vi "Actor Core.vi"(8 "error in (no error)":errorcluster, 11 "Operator UI.lvclass":refnum<class "Server UI.lvclass">) -> (0 "error out":errorcluster, 3 "Actor Framework.lvlib:Actor":refnum<class "Actor.lvclass">)   [LabVIEW 2017, in "Server UI.lvlib" / "Server UI.lvclass"]
doc: "This is Actor Core.vi, the main message handling loop for Actors. An actor usually just sits in this loop and processes messages as they arrive. Any error returned by the message Do.vi call will stop the loop, with error code 43 as the cannonical signal to stop with no error sent to caller. Descendants may override that in Handle Error.vi."
uses:
  Server UI.lvclass
  <vilib>/ActorFramework/Actor/Actor.lvclass
  \\Mac\Home/Documents/MAL-Framework/user.lib/Common Components/Msmt UI/Measurement UI.lvclass
  \\Mac\Home/Documents/MAL-Framework/user.lib/Common Components/User Interface/UI.lvclass
  C:/Program Files (x86)/National Instruments/LabVIEW 2017/vi.lib/ActorFramework/Actor/Actor.lvclass
  Server UI.lvclass/Server UI.ctl
  <vilib>/ActorFramework/Actor/Actor.lvclass/Actor.ctl
  <vilib>/ActorFramework/Message Enqueuer/Message Enqueuer.lvclass/Message Enqueuer.ctl
  Write Start Server.vi
  Write Connected Clients.vi
  <vilib>/ActorFramework/Message Enqueuer/Init from Existing Queue.vi
  <vilib>/ActorFramework/Message Enqueuer/Enqueue.vi
  <vilib>/ActorFramework/Stop Msg/Stop Msg.lvclass
  C:/Program Files (x86)/National Instruments/LabVIEW 2017/vi.lib/ActorFramework/Message/Message.lvclass
  MAL-Framework/user.lib/Common Components/User Interface/Messages/Disable UI Msg/Disable UI Msg.lvclass
  Server UI Messages/Show Connections Msg/Show Connections Msg.lvclass
  MAL-Framework/user.lib/Common Components/Msmt UI/Messages/Ask Controller to Launch Results UI Msg/Ask Controller to Launch Results UI Msg.lvclass
  MAL-Framework/user.lib/Common Components/User Interface/Messages/Reset Controls Msg/Reset Controls Msg.lvclass
  Server UI Messages/Reset Measurement List Display Msg/Reset Measurement List Display Msg.lvclass
  MAL-Framework/user.lib/Common Components/Measurement UI Messages/Launch Step Configuration Msg/Launch Step Configuration Msg.lvclass
  MAL-Framework/user.lib/Common Components/User Interface/Messages/Enable UI Msg/Enable UI Msg.lvclass
  MAL-Framework/user.lib/Common Components/Msmt UI/Messages/Tell Controller to Launch Settings Dialog Msg/Tell Controller to Launch Settings Dialog Msg.lvclass
  MAL-Framework/user.lib/Common Components/Msmt UI/Accessors/Write Digitizer.vi
  MAL-Framework/user.lib/Common Components/Msmt UI/Accessors/Write Function Generator.vi
  MAL-Framework/user.lib/Common Components/Msmt UI/Accessors/Write Load New Measurement.vi
  MAL-Framework/user.lib/Common Components/Msmt UI/Accessors/Write Measurement.vi
  MAL-Framework/user.lib/Common Components/Msmt UI/Accessors/Write Multimeter.vi
  MAL-Framework/user.lib/Common Components/Msmt UI/Accessors/Write Power Supply.vi
  MAL-Framework/user.lib/Common Components/Msmt UI/Accessors/Write Results Listbox.vi
  MAL-Framework/user.lib/Common Components/Msmt UI/Accessors/Write Run.vi
  MAL-Framework/user.lib/Common Components/Msmt UI/Accessors/Write Show FP_.vi
  MAL-Framework/user.lib/Common Components/Msmt UI/Accessors/Write Status Display.vi
  MAL-Framework/user.lib/Common Components/Msmt UI/Accessors/Write Tab Control.vi
  MAL-Framework/user.lib/Common Components/Msmt UI/Accessors/Write View Results.vi
  MAL-Framework/user.lib/Common Components/User Interface/Accessors/Write Settings Button.vi
  MAL-Framework/user.lib/Common Components/Msmt UI/Accessors/Write Run Indefinitely.vi
  MAL-Framework/user.lib/Common Components/Msmt UI/Write Step Iterations.vi
  MAL-Framework/user.lib/Common Components/Msmt UI/Write settings button array for hardware.vi
  MAL-Framework/user.lib/Common Components/Msmt UI/Accessors/Write Step Config.vi
  <vilib>/ActorFramework/Message Priority Queue/Priority Enqueue.vi
  <vilib>/ActorFramework/Message Enqueuer/Message Enqueuer.lvclass
  MAL-Framework/user.lib/Common Components/Msmt UI/Measurement UI.lvclass
  MAL-Framework/user.lib/Common Components/Msmt UI/Messages/Send Run Measurement Message/Send Run Measurement Message.lvclass
  MAL-Framework/user.lib/Common Components/Msmt UI/Messages/Send Get Hardware Info Message/Send Get Hardware Info Message.lvclass
  MAL-Framework/user.lib/Common Components/Msmt UI/Messages/Check Run Button/Check Validity of Selection.lvclass
  MAL-Framework/user.lib/Common Components/Msmt UI/Messages/Prompt User for Path to load/Prompt User for File Path to Load From.lvclass
  MAL-Framework/user.lib/Common Components/User Interface/UI.lvclass
  MAL-Framework/user.lib/Common Components/Measurement UI Messages/Launch Hardware Settings Msg/Launch Hardware Settings Msg.lvclass
panel:
  in  "Connected Clients":i32(listbox)
  in  "Step Config":bool
  in  "3":bool
  in  "2":bool
  in  "1":bool
  in  "0":bool
  in  "Step Iterations":i32
  in  "Run Indefinitely":bool
  in  "Show FP?":bool
  in  "Power Supply":u16(ring) caption="4"
  in  "Function Generator":u16(ring) caption="3"
  in  "Digitizer":u16(ring) caption="2"
  in  "Multimeter":u16(ring) caption="1"
  in  "Step":u16(ring)
  in  "about":bool
  in  "Tab Control":enum32{"Test Status", "Results"}(tab)
  in  "Status Display":string
  in  "View Results":bool
  in  "Results Listbox":i32(listbox)
  in  "Settings Button":bool
  in  "Start Server":bool
  in  "Load New Measurement":bool
  in  "Run":bool
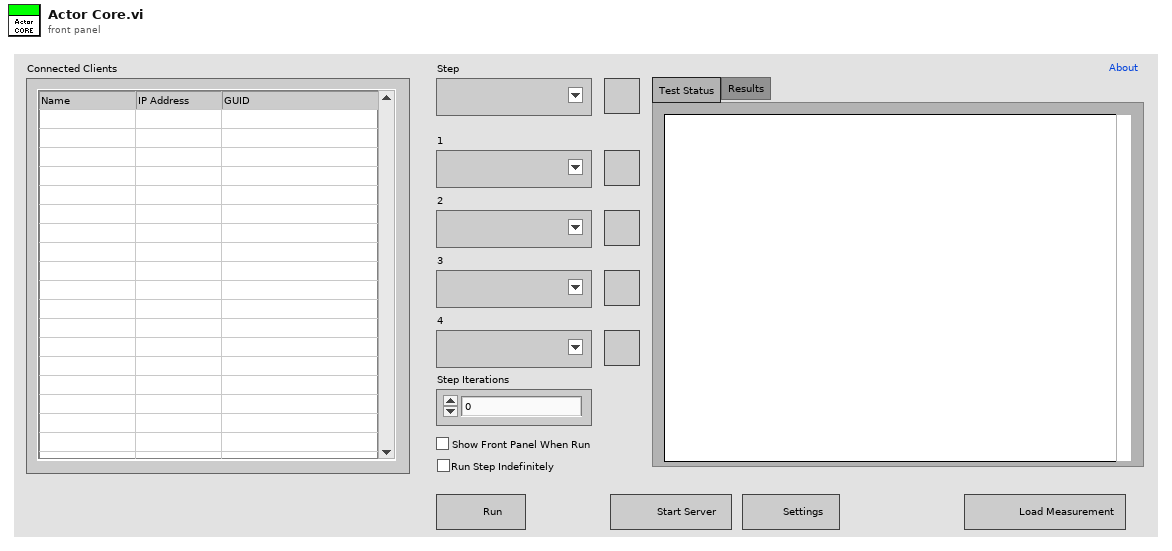
[diagram p1: front panel]
types:
  T1 = enum8{"Enabled", "Disabled", "Disabled and Grayed Out"}
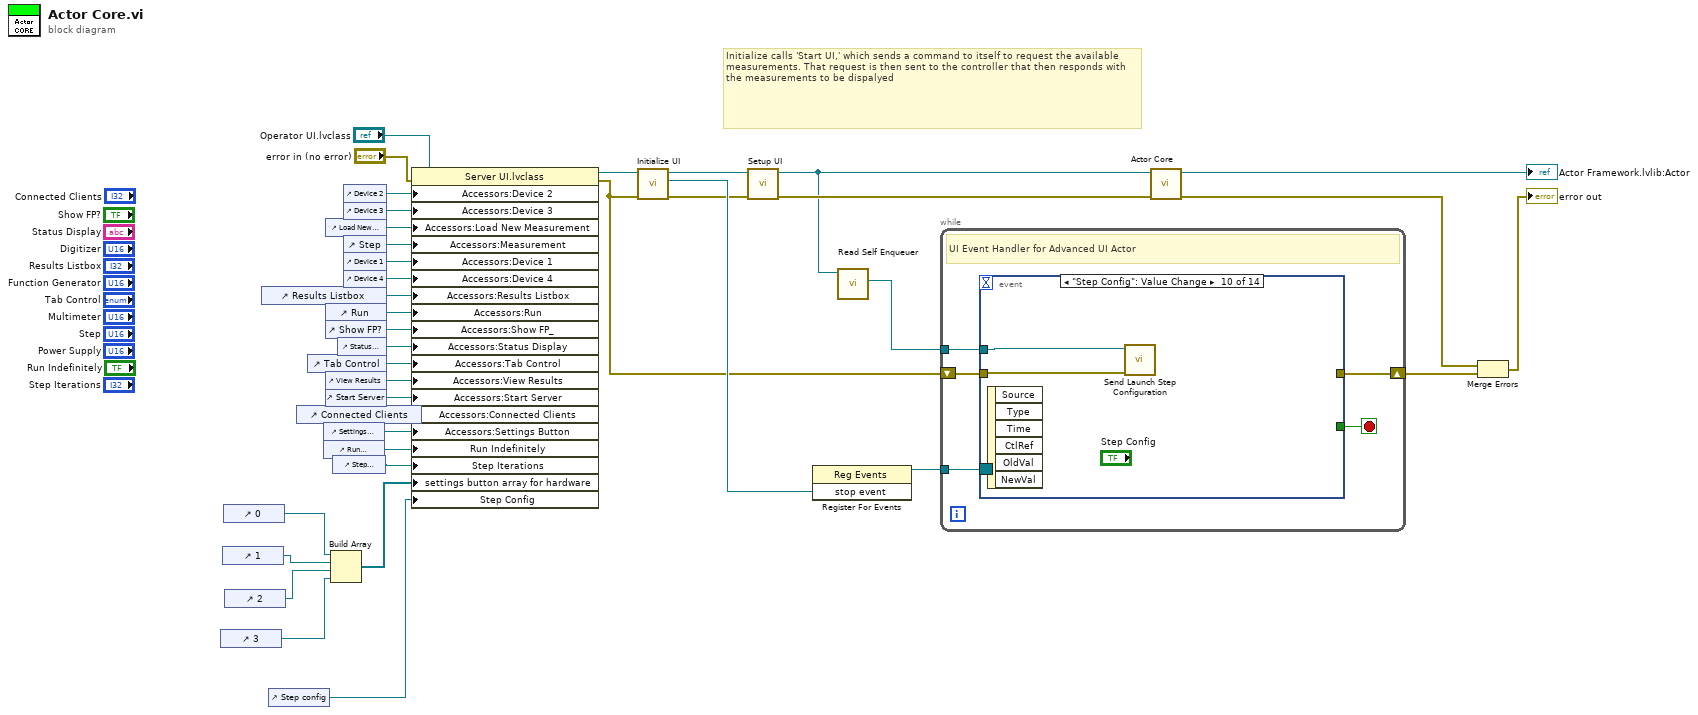
[diagram p0: block diagram]
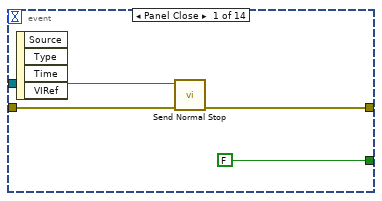
[diagram p2: hidden frame]
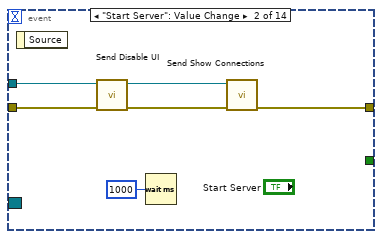
[diagram p3: hidden frame]
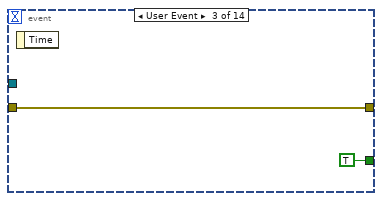
[diagram p4: hidden frame]
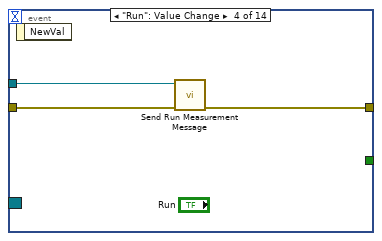
[diagram p5: hidden frame]
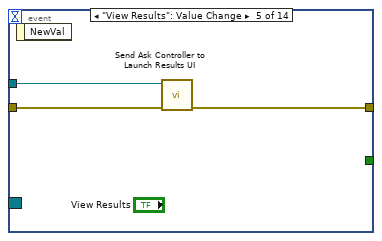
[diagram p6: hidden frame]
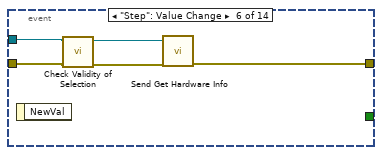
[diagram p7: hidden frame]
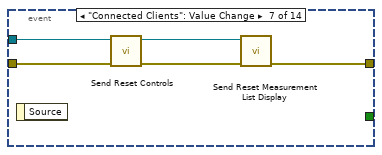
[diagram p8: hidden frame]
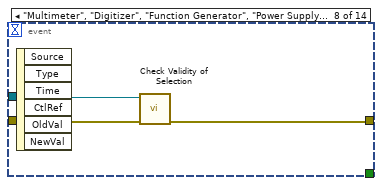
[diagram p9: hidden frame]
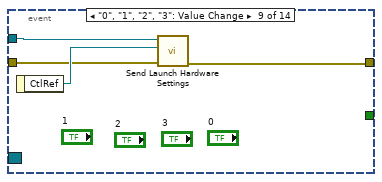
[diagram p10: hidden frame]
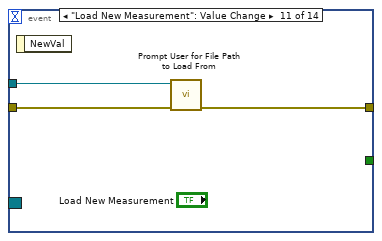
[diagram p11: hidden frame]
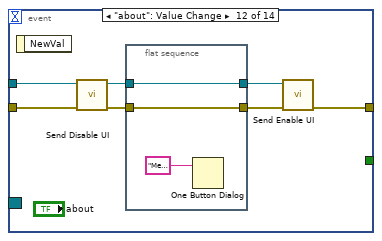
[diagram p12: hidden frame]
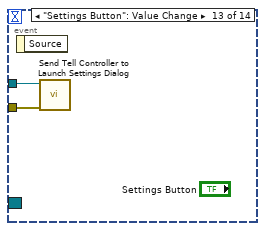
[diagram p13: hidden frame]
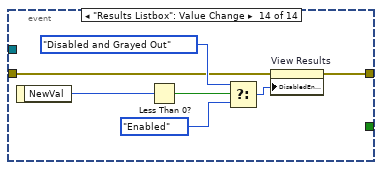
[diagram p14: hidden frame]
diagram:
  # "Initialize calls 'Start UI,' which sends a command to itself to request the available measurements. That request is then sent to the controller that then responds with the measurements to be dispalyed"
  n1 = control-ref of="3"() -> (w6:refnum<vi>)
  n2 = control-ref of="1"() -> (w4:refnum<vi>)
  n3 = control-ref of="0"() -> (w3:refnum<vi>)
  n4 = control-ref of="2"() -> (w5:refnum<vi>)
  n5 = control-ref of="Results Listbox"() -> (w29:refnum<vi>)
  n6 = control-ref of="Step config"() -> (w1:refnum<vi>)
  n7 = control-ref of="Connected Clients"() -> (w11:refnum<vi>)
  n8 = control-ref of="Tab Control"() -> (w31:refnum<vi>)
  n9 = control-ref of="Settings Button"() -> (w9:refnum<vi>)
  n10 = control-ref of="Run Indefinitely"() -> (w8:refnum<vi>)
  n11 = control-ref of="Load New Measurement"() -> (w25:refnum<vi>)
  n12 = control-ref of="Run"() -> (w22:refnum<vi>)
  n13 = control-ref of="Show FP?"() -> (w33:refnum<vi>)
  n14 = control-ref of="View Results"() -> (w30:refnum<vi>)
  n15 = control-ref of="Start Server"() -> (w12:refnum<vi>)
  n16 = Build Array(w3, w4, w5, w6) -> (w2:refnum<vi>[])
  n17 = control-ref of="Step Iterations"() -> (w7:refnum<vi>)
  n18 = control-ref of="Status Display"() -> (w32:refnum<vi>)
  n19 = control-ref of="Device 2"() -> (w27:refnum<vi>)
  n20 = control-ref of="Device 3"() -> (w26:refnum<vi>)
  n21 = control-ref of="Step"() -> (w24:refnum<vi>)
  n22 = control-ref of="Device 1"() -> (w23:refnum<vi>)
  n23 = control-ref of="Device 4"() -> (w28:refnum<vi>)
  n24 = property class="Server UI.lvclass"(reference="Operator UI.lvclass", error in="error in (no error)", "Accessors:Device 2"=w27, "Accessors:Device 3"=w26, "Accessors:Load New Measurement"=w25, "Accessors:Measurement"=w24, "Accessors:Device 1"=w23, "Accessors:Device 4"=w28, "Accessors:Results Listbox"=w29, "Accessors:Run"=w22, "Accessors:Show FP_"=w33, "Accessors:Status Display"=w32, "Accessors:Tab Control"=w31, "Accessors:View Results"=w30, "Accessors:Start Server"=w12, "Accessors:Connected Clients"=w11, "Accessors:Settings Button"=w9, "Run Indefinitely"=w8, "Step Iterations"=w7, "settings button array for hardware"=w2, "Step Config"=w1) -> (reference out=w17:refnum<class "Server UI.lvclass">, error out=w14:errorcluster)
  n25 = call "Initialize UI.vi"("error in (no error)"=w14, "UI in"=w17) -> ("error out"=w13:errorcluster, "stop event"=w34:refnum<user-event>, "UI out"=w16:refnum<class "Server UI.lvclass">)  [unwired: 7 in]
  n26 = call-dynamic "Setup UI.vi"("error in (no error)"=w13, "Operator UI in"=w16) -> ("error out"=w15:errorcluster, "Operator UI out"=w10:refnum<class "Server UI.lvclass">)  [unwired: 8 in]
  n27 = register-events(w34) -> (reference out=w35:refnum<event-registration>)  [unwired: 2 in, 1 out]
  n28 = call <vilib>:"Read Self Enqueuer.vi"("Actor"=w10) -> ("Self Enqueuer"=w37:refnum<class "Message Enqueuer.lvclass">)  [unwired: 10 in]
  n29 = while {
    tunnel: w37 -> [w42]
    tunnel: w35 -> [w41]
    shift-right: [w39] -> w36
    shift-left: w14 -> [w40]
    stop <- w43 stop-if-true
    # "UI Event Handler for Advanced UI Actor"
    n30 = event shown="[9] \"Step Config\": Value Change" {
      selector: w41 -> [_ _ _ _ _ _ _ _ _ _ _ _ _ _]
      dyn-events: _ -> [_ _ _ _ _ _ _ _ _ _ _ _ _ _]
      timeout: _ -> [_ _ _ _ _ _ _ _ _ _ _ _ _ _]
      tunnel: [FALSE _ TRUE _ _ _ _ _ _ _ _ _ _ _] -> w43
      tunnel: w42 -> [w46 w51 _ w58 w61 w65 w71 w74 w78 w80 w83 w90 w94 _]
      tunnel: w40 -> [w45 w50 w54 w57 w60 w64 w70 w73 w76 w79 w82 w89 w95 w97]
      tunnel: [w44 w48 w54 w56 w59 w66 w67 w72 w75 _ w81 w84 _ w96] -> w39
      event Panel Close {
        n31 = event-data() -> ()  [unwired: 1 in, 4 out]
        n32 = call <vilib>:"Send Normal Stop.vi"("error in (no error)"=w45, "Message Enqueuer"=w46) -> ("error out"=w44:errorcluster)  [unwired: 9 in]
      }
      event "Start Server": Value Change {
        n33 = event-data() -> ()  [unwired: 1 in, 1 out]
        n34 = call "Send Disable UI.vi"("error in (no error)"=w50, "Message Enqueuer"=w51) -> ("error out"=w49:errorcluster, "Message Enqueuer out"=w52:refnum<class "Message Enqueuer.lvclass">)  [unwired: 8 in]
        n35 = Wait (ms)(milliseconds to wait=u32 1000) -> ()  [unwired: 1 out]
        n36 = call "Send Show Connections.vi"("error in (no error)"=w49, "Message Enqueuer"=w52) -> ("error out"=w48:errorcluster)  [unwired: 8 in, 1 out]
      }
      event User Event {
        n37 = event-data() -> ()  [unwired: 1 in, 1 out]
      }
      event "Run": Value Change {
        n38 = event-data() -> ()  [unwired: 1 in, 1 out]
        n39 = call "Send Run Measurement Message.vi"("error in (no error)"=w57, "Message Enqueuer in"=w58) -> ("error out"=w56:errorcluster)  [unwired: 8 in, 1 out]
      }
      event "View Results": Value Change {
        n40 = event-data() -> ()  [unwired: 1 in, 1 out]
        n41 = call "Send Ask Controller to Launch Results UI.vi"("error in (no error)"=w60, "Message Enqueuer in"=w61) -> ("error out"=w59:errorcluster)  [unwired: 8 in, 1 out]
      }
      event "Step": Value Change {
        n42 = event-data() -> ()  [unwired: 1 in, 1 out]
        n43 = call "Check Validity of Selection.vi"("error in (no error)"=w64, "Message Enqueuer in"=w65) -> ("error out"=w63:errorcluster, "Message Enqueuer out"=w62:refnum<class "Message Enqueuer.lvclass">)  [unwired: 8 in]
        n44 = call "Send Get Hardware Info.vi"("error in (no error)"=w63, "Message Enqueuer in"=w62) -> ("error out"=w66:errorcluster)  [unwired: 8 in, 1 out]
      }
      event "Connected Clients": Value Change {
        n45 = event-data() -> ()  [unwired: 1 in, 1 out]
        n46 = call "Send Reset Controls.vi"("error in (no error)"=w70, "Message Enqueuer"=w71) -> ("error out"=w68:errorcluster, "Message Enqueuer out"=w69:refnum<class "Message Enqueuer.lvclass">)  [unwired: 8 in]
        n47 = call "Send Reset Measurement List Display.vi"("error in (no error)"=w68, "Message Enqueuer"=w69) -> ("error out"=w67:errorcluster)  [unwired: 8 in, 1 out]
      }
      event "Multimeter", "Digitizer", "Function Generator", "Power Supply", "Step Iterations", "Run Indefinitely": Value Change {
        n48 = event-data() -> ()  [unwired: 1 in, 6 out]
        n49 = call "Check Validity of Selection.vi"("error in (no error)"=w73, "Message Enqueuer in"=w74) -> ("error out"=w72:errorcluster)  [unwired: 8 in, 1 out]
      }
      event "0", "1", "2", "3": Value Change {
        n50 = event-data() -> ("CtlRef"=w77:refnum<vi>)  [unwired: 1 in]
        n51 = call "Send Launch Hardware Settings.vi"("error in (no error)"=w76, "button ref"=w77, "Message Enqueuer"=w78) -> ("error out"=w75:errorcluster)  [unwired: 7 in, 1 out]
      }
      event "Step Config": Value Change {
        n52 = event-data() -> ()  [unwired: 1 in, 6 out]
        n53 = call "Send Launch Step Configuration.vi"("error in (no error)"=w79, "Message Enqueuer"=w80) -> ()  [unwired: 8 in, 2 out]
      }
      event "Load New Measurement": Value Change {
        n54 = event-data() -> ()  [unwired: 1 in, 1 out]
        n55 = call "Prompt User for File Path to Load From.vi"("error in (no error)"=w82, "Message Enqueuer in"=w83) -> ("error out"=w81:errorcluster)  [unwired: 8 in, 1 out]
      }
      event "about": Value Change {
        n56 = event-data() -> ()  [unwired: 1 in, 1 out]
        n57 = call "Send Disable UI.vi"("error in (no error)"=w89, "Message Enqueuer"=w90) -> ("error out"=w88:errorcluster, "Message Enqueuer out"=w86:refnum<class "Message Enqueuer.lvclass">)  [unwired: 8 in]
        n58 = flat-sequence {
          tunnel: [w92] -> w87
          tunnel: w88 -> [w92]
          tunnel: [w91] -> w85
          tunnel: w86 -> [w91]
          frame #0 {
            n59 = One Button Dialog(message="Measurement Manager v3.0 ALPHA RELEASE\n\nNational Instruments (C) 2013\nWritten in NI LabVIEW 2013 by Elijah Kerry \nElijah.Kerry@ni.com\n\nekerry.wordpress.com\nLatest version: bit.ly/lv_oomal") -> ()  [unwired: 1 in, 1 out]
          }
        }
        n60 = call "Send Enable UI.vi"("error in (no error)"=w87, "Message Enqueuer"=w85) -> ("error out"=w84:errorcluster)  [unwired: 8 in, 1 out]
      }
      event "Settings Button": Value Change {
        n61 = event-data() -> ()  [unwired: 1 in, 1 out]
        n62 = call "Send Tell Controller to Launch Settings Dialog.vi"("error in (no error)"=w95, "Message Enqueuer"=w94) -> ()  [unwired: 8 in, 2 out]
      }
      event "Results Listbox": Value Change {
        n63 = event-data() -> ("NewVal"=w98:i32)  [unwired: 1 in]
        n64 = Less Than 0?(x=w98) -> (x < 0?=w99:bool)
        n65 = Select(t=T1."Disabled and Grayed Out" ("Disabled"), s=w99, f=T1."Enabled" ("Disabled")) -> (s? t:f=w102:T1)
        n66 = property on="View Results" class="Bool"(error in=w97, "DisabledEnum"=w102) -> (error out=w96:errorcluster)  [unwired: 1 in, 1 out]
      }
    }
  }
  n67 = call-parent "Actor Core.vi"("error in (no error)"=w15, "Operator UI.lvclass"=w10) -> ("error out"=w20:errorcluster, "Actor Framework.lvlib:Actor"=→"Actor Framework.lvlib:Actor":refnum<class "Actor.lvclass">)  [unwired: 8 in]
  n68 = Merge Errors(w20, w36) -> (→"error out":errorcluster)
